vi "autoNode.vi"(6 "Variant in":variant, 7 "Shift Pressed?":bool, 8 "error in (no error)":errorcluster, 10 "QD Combo Box Ref":refnum<vi>, 11 "QD Launch VI Ref":refnum<vi>) -> (0 "error out":errorcluster, 4 "Variant out":variant)   [LabVIEW 2015]
doc: "Base controls to distribute nodes in panel.\n\nDefault Shortcut - [G]"
panel:
  in  "Undo Name":string="Dup Con I/O"
  # "Do not change the connector pane of this VI.\n\nSee the block diagram for directions on how to use this template."
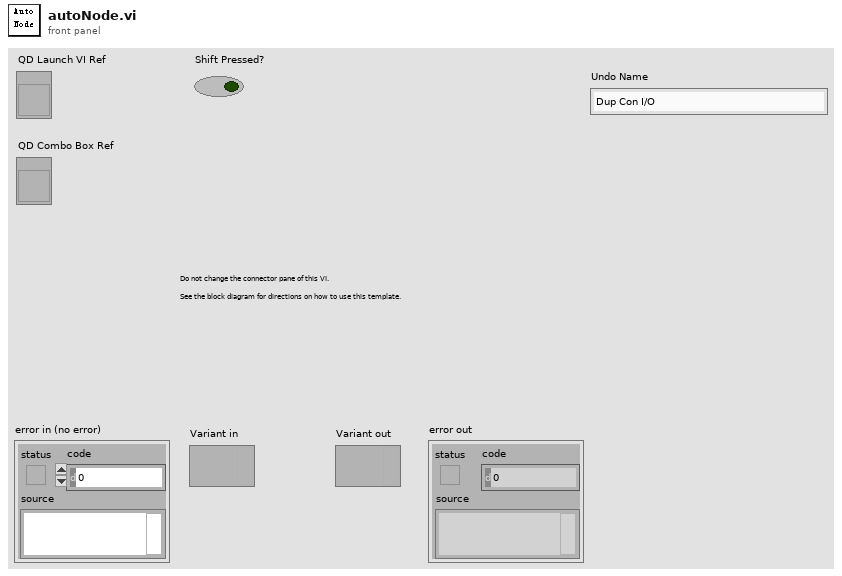
[diagram p1: front panel]
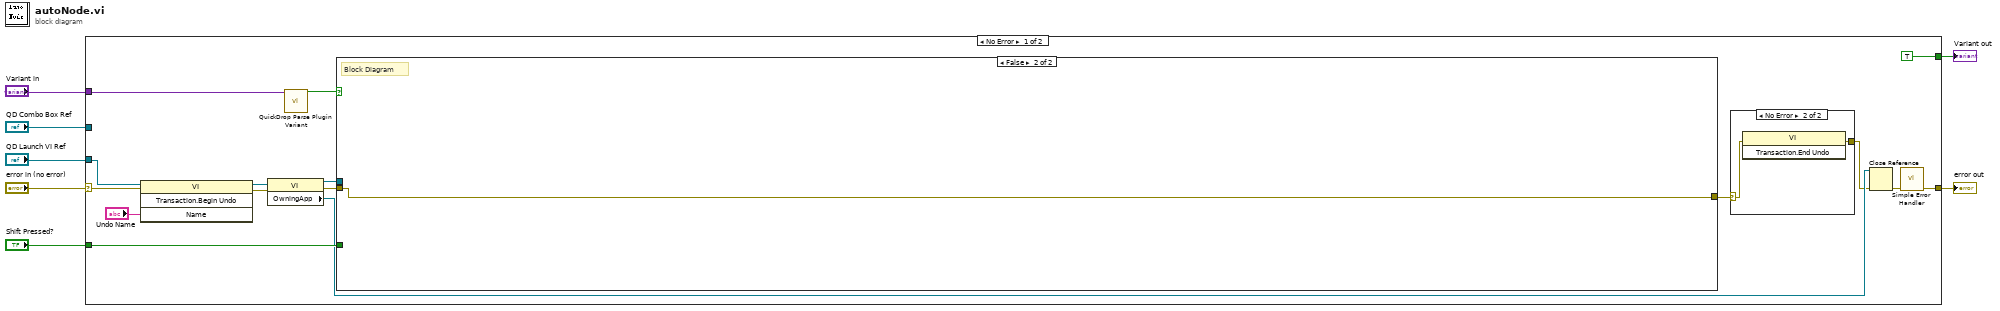
[diagram p0: block diagram]
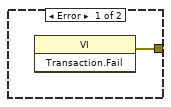
[diagram p2: hidden frame]
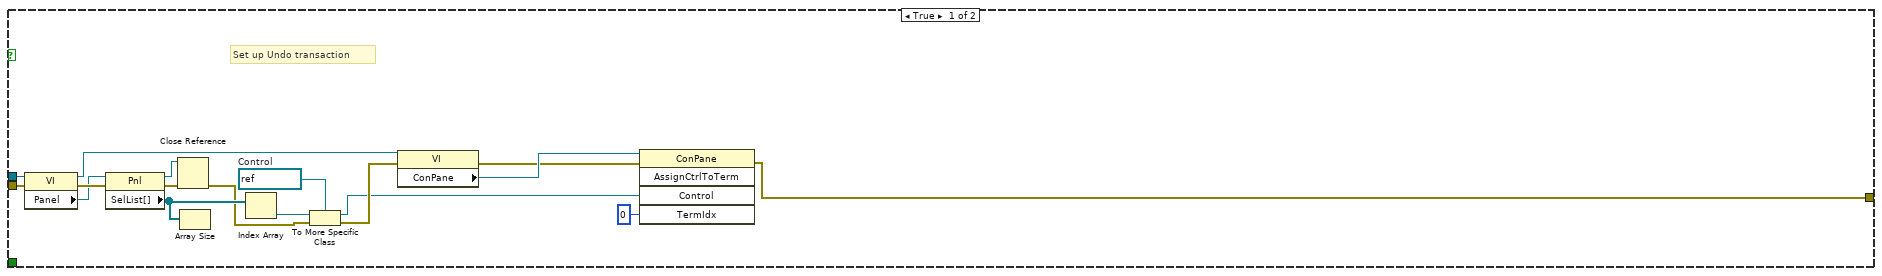
[diagram p3: hidden frame]
diagram:
  n1 = case shown="No Error" "error in (no error)" {
    selector: "error in (no error)" -> [w11 w45]
    tunnel: [w16 w45] -> w6
    tunnel: "QD Launch VI Ref" -> [w13 _]
    tunnel: "Shift Pressed?" -> [w21 _]
    tunnel: "QD Combo Box Ref" -> [_ _]
    tunnel: "Variant in" -> [w23 _]
    tunnel: [TRUE _] -> w1
    frame No Error {
      n2 = invoke class="VI" method="Transaction.Begin Undo"(reference=w13, error in=w11, "Name"="Undo Name") -> (reference out=w12:refnum<vi>, error out=w10:errorcluster)  [unwired: 1 in, 2 out]
      n3 = property class="VI"(reference=w12, error in=w10) -> (reference out=w19:refnum<vi>, error out=w18:errorcluster, "OwningApp"=w15:refnum<vi>)
      n4 = call <vilib>:"QuickDrop Parse Plugin Variant.vi"("QDKS Variant in"=w23) -> ("QD Launch VI Panel?"=w20:bool)  [unwired: 12 in, 2 out]
      n5 = case shown="False" w20 {
        tunnel: w18 -> [w43 w44]
        tunnel: w21 -> [_ _]
        tunnel: w19 -> [w42 _]
        tunnel: [w27 w44] -> w8
        frame True {
          w35 = refnum<vi> refnum  # Control
          # "Set up Undo transaction"
          n6 = property class="VI"(reference=w42, error in=w43) -> (reference out=w33:refnum<vi>, error out=w41:errorcluster, "Panel"=w40:refnum<vi>)
          n7 = property class="Pnl"(reference=w40, error in=w41) -> (reference out=w39:refnum<vi>, error out=w38:errorcluster, "SelList[]"=w37:refnum<vi>[])
          n8 = Close Reference(reference=w39, error in (no error)=w38) -> (error out=w34:errorcluster)
          n9 = Array Size(array=w37) -> ()  [unwired: 1 out]
          n10 = Index Array(array=w37) -> (element=w36:refnum<vi>)  [unwired: 1 in]
          n11 = To More Specific Class(target class=w35, reference=w36, error in=w34) -> (specific class reference=w30:refnum<vi>, error out=w32:errorcluster)
          n12 = property class="VI"(reference=w33, error in=w32) -> (error out=w28:errorcluster, "ConPane"=w31:refnum<vi>)  [unwired: 1 out]
          n13 = invoke class="ConPane" method="AssignCtrlToTerm"(reference=w31, error in=w28, "Control"=w30, "TermIdx"=u32 0 ("Terminal Index")) -> (error out=w27:errorcluster)  [unwired: 1 in, 4 out]
        }
        frame False {
          # "Block Diagram"
        }
      }
      n14 = case shown="No Error" w8 {
        selector: w8 -> [_ w25]
        tunnel: [w24 w26] -> w9
        frame Error {
          n15 = invoke class="VI" method="Transaction.Fail"() -> (error out=w24:errorcluster)  [unwired: 3 in, 2 out]
        }
        frame No Error {
          n16 = invoke class="VI" method="Transaction.End Undo"(error in=w25) -> (error out=w26:errorcluster)  [unwired: 2 in, 2 out]
        }
      }
      n17 = Close Reference(reference=w15, error in (no error)=w9) -> (error out=w17:errorcluster)
      n18 = call <vilib>:"Simple Error Handler.vi"("error in (no error)"=w17) -> ("error out"=w16:errorcluster)  [unwired: 4 in, 4 out]
    }
    frame Error {
    }
  }
  "error out" <- w6
  "Variant out" <- w1
